vi "FGV Interference.vi"(0 "TestKonfig":T5={"CH4:"=0, "Ethane:"=0, "NMHC:"=0, "NMNEHC:"=0, "Komp 1 aktiv:"=FALSE, "Komp 2 aktiv:"=FALSE, "Komp 3 aktiv:"=FALSE, "Komp 4 aktiv:"=FALSE, "Modus"=0, "CG Aufschaltzeit:"=120.0, "Interferent 1: CO2"=0, "Interferent 2: H2O"=0, "Interferent 3: CH4"=0, "Interferent 4: C2H6 / C3H8"=0, "Gasflaschen Nr.:"="", "Gasflaschen Nr.: 3"="", "Gasflaschen Nr.: 4"="", "Inter 1 aktiv"=FALSE, "Inter 2 aktiv"=FALSE, "Inter 3 aktiv"=FALSE, "Inter 4 aktiv"=FALSE, "Accuracy"="", "Accuracy 3"="", "Accuracy 4"="", "Konzentration 1:"=120.0, "Konzentration 2:"=120.0, "Konzentration 3:"=120.0, "Konzentration 4:"=120.0, "Flow weighted mean 1:"=0.0, "Flow weighted mean 2:"=0.0, "Flow weighted mean 3:"=0.0, "Flow weighted mean 4:"=0.0} {"Flow weighted mean 4:" min=0.0; "Flow weighted mean 3:" min=0.0; "Flow weighted mean 2:" min=0.0; "Flow weighted mean 1:" min=0.0; "Konzentration 4:" min=0.0; "Konzentration 3:" min=0.0; "Konzentration 2:" min=0.0; "Konzentration 1:" min=0.0; "Modus" items=["Messen", "CG zu Entnahmestelle"]; "CG Aufschaltzeit:" min=60.0}, 1 "TestSetting":T1={"Bearbeiter:"="", "Pfad:"=path "D:/IAG_Data/Log", "Textname:"="", "Analysator"=""}, 5 "Ergebnis":sgl[](array[numeric]), 7 "Êinheiten":string[](array[string]), 9 "Tabelle":T3[][](array[typedef]), 11 "error in (no error)":errorcluster caption="Fehler (Eingang, kein Fehler)", 12 "Aktion FGV Interference":T7) -> (3 "TestSetting":T1={"Bearbeiter:"="", "Pfad:"=path "D:/IAG_Data/Log", "Textname:"="", "Analysator"=""}, 4 "TestKonfig":T5={"CH4:"=0, "Ethane:"=0, "NMHC:"=0, "NMNEHC:"=0, "Komp 1 aktiv:"=FALSE, "Komp 2 aktiv:"=FALSE, "Komp 3 aktiv:"=FALSE, "Komp 4 aktiv:"=FALSE, "Modus"=0, "CG Aufschaltzeit:"=120.0, "Interferent 1: CO2"=0, "Interferent 2: H2O"=0, "Interferent 3: CH4"=0, "Interferent 4: C2H6 / C3H8"=0, "Gasflaschen Nr.:"="", "Gasflaschen Nr.: 3"="", "Gasflaschen Nr.: 4"="", "Inter 1 aktiv"=FALSE, "Inter 2 aktiv"=FALSE, "Inter 3 aktiv"=FALSE, "Inter 4 aktiv"=FALSE, "Accuracy"="", "Accuracy 3"="", "Accuracy 4"="", "Konzentration 1:"=120.0, "Konzentration 2:"=120.0, "Konzentration 3:"=120.0, "Konzentration 4:"=120.0, "Flow weighted mean 1:"=0.0, "Flow weighted mean 2:"=0.0, "Flow weighted mean 3:"=0.0, "Flow weighted mean 4:"=0.0} {"Flow weighted mean 4:" min=0.0; "Flow weighted mean 3:" min=0.0; "Flow weighted mean 2:" min=0.0; "Flow weighted mean 1:" min=0.0; "Konzentration 4:" min=0.0; "Konzentration 3:" min=0.0; "Konzentration 2:" min=0.0; "Konzentration 1:" min=0.0; "Modus" items=["Messen", "CG zu Entnahmestelle"]; "CG Aufschaltzeit:" min=60.0}, 6 "Ergebnis":T4, 8 "Êinheiten":string[](array[string]), 10 "Tabelle":T3[][](array[typedef]), 15 "error out":errorcluster caption="Fehler (Ausgang)")   [LabVIEW 2020, in "EPA 1065.lvlib" / "Interference verificaton 1065-366.lvlib"]
uses:
  Interference verificaton 1065-366.lvlib
  Aktion FGV Interference.ctl
  TestKonfig.ctl
  Modus.ctl
  Ergebnis.ctl
  Visualisierungs Elemente/String - Ausgabefeld.ctl
  TestSetting.ctl
  Seiten/System Einstellungen V2/Analysatoren.ctl
  Linearisierung V2/AktivButton.ctl
  Allgemein/allgemeine Sub-VIs.lvlib
  Linearisierung V2/Linearisierung v2.lvlib
  Seiten/System Einstellungen V2/System Einstellungen V2.lvlib
panel:
  in  "Ergebnis":T4 caption="Cluster"
  # "sec."
  # "sec."
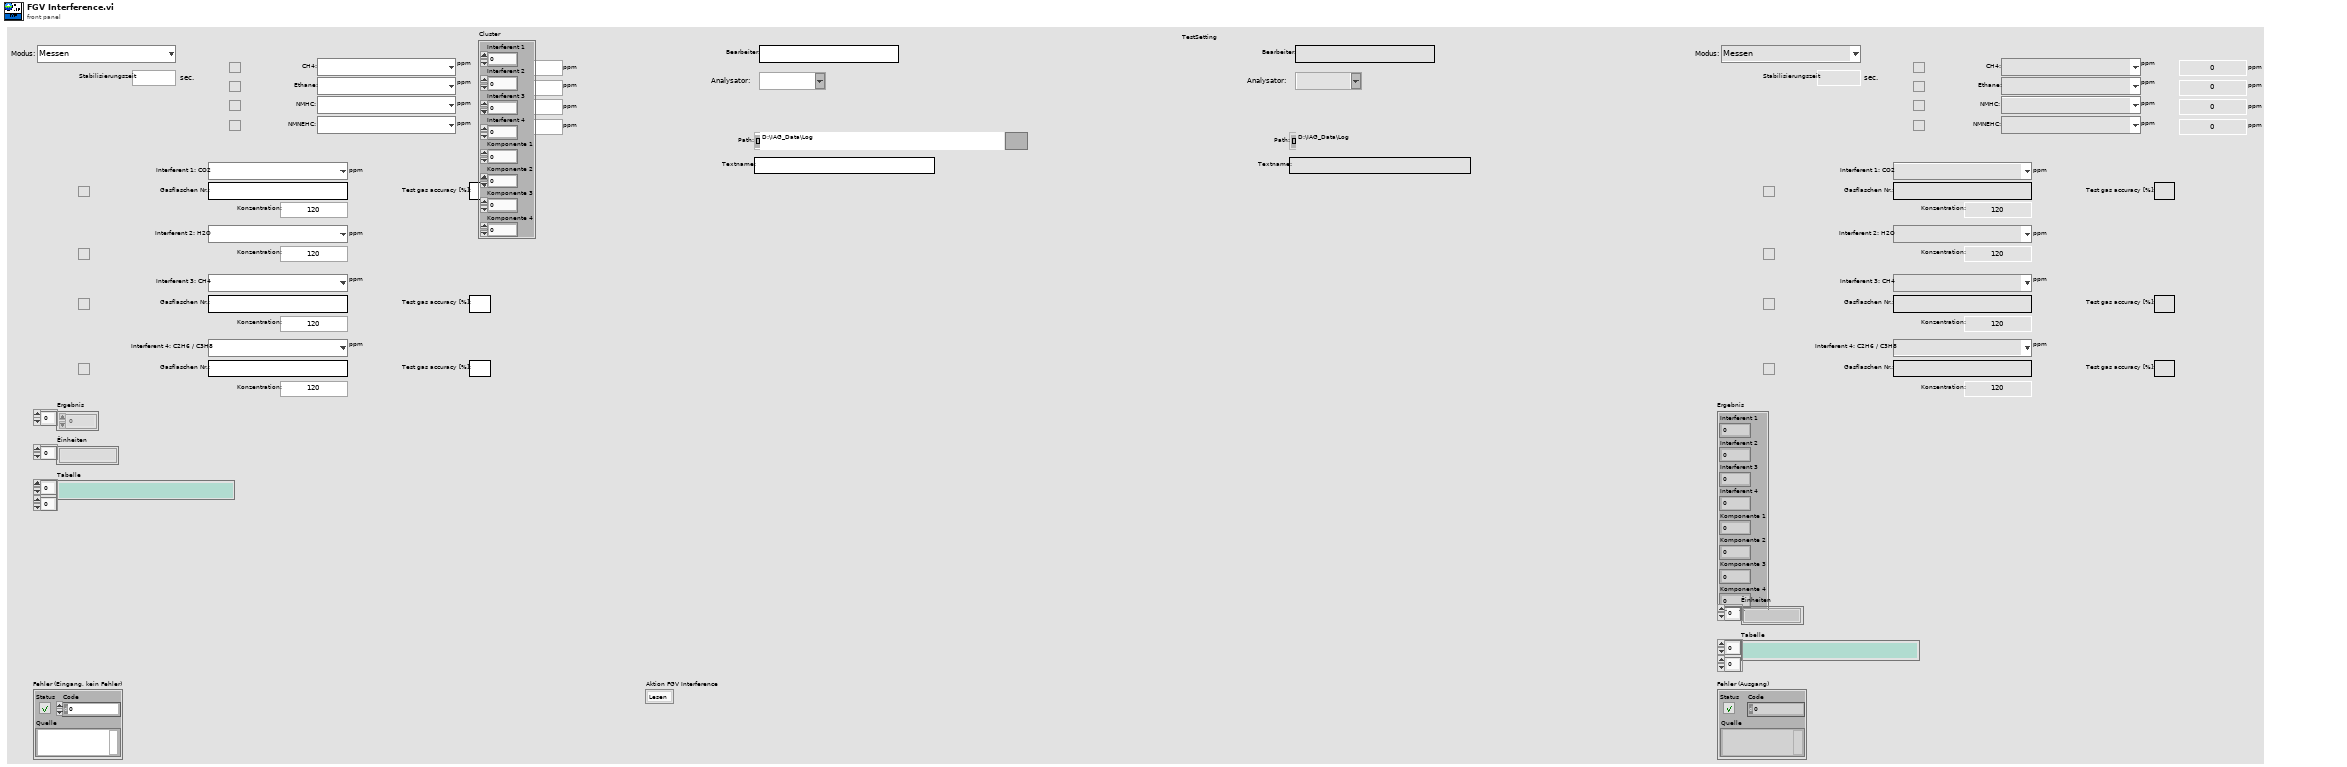
[diagram p1: front panel]
types:
  T1 = typedef "EPA 1065.lvlib/Interference verificaton 1065-366.lvlib/TestSetting.ctl" = cluster{"Bearbeiter:":string, "Pfad:":path, "Textname:":string, "Analysator":T2}
  T2 = typedef "System Einstellungen V2.lvlib/Analysatoren.ctl" = string
  T3 = typedef "String - Ausgabefeld.ctl" = string
  T4 = typedef "EPA 1065.lvlib/Interference verificaton 1065-366.lvlib/Ergebnis.ctl" = cluster{"Interferent 1":sgl, "Interferent 2":sgl, "Interferent 3":sgl, "Interferent 4":sgl, "Komponente 1":sgl, "Komponente 2":sgl, "Komponente 3":sgl, "Komponente 4":sgl}
  T5 = typedef "EPA 1065.lvlib/Interference verificaton 1065-366.lvlib/TestKonfig.ctl" = cluster{"CH4:":u16, "Ethane:":u16, "NMHC:":u16, "NMNEHC:":u16, "Komp 1 aktiv:":bool, "Komp 2 aktiv:":bool, "Komp 3 aktiv:":bool, "Komp 4 aktiv:":bool, "Modus":T6, "CG Aufschaltzeit:":dbl, "Interferent 1: CO2":u16, "Interferent 2: H2O":u16, "Interferent 3: CH4":u16, "Interferent 4: C2H6 / C3H8":u16, "Gasflaschen Nr.:":string, "Gasflaschen Nr.: 3":string, "Gasflaschen Nr.: 4":string, "Inter 1 aktiv":bool, "Inter 2 aktiv":bool, "Inter 3 aktiv":bool, "Inter 4 aktiv":bool, "Accuracy":string, "Accuracy 3":string, "Accuracy 4":string, "Konzentration 1:":dbl, "Konzentration 2:":dbl, "Konzentration 3:":dbl, "Konzentration 4:":dbl, "Flow weighted mean 1:":dbl, "Flow weighted mean 2:":dbl, "Flow weighted mean 3:":dbl, "Flow weighted mean 4:":dbl}
  T6 = typedef "EPA 1065.lvlib/Interference verificaton 1065-366.lvlib/Modus.ctl" = u16
  T7 = typedef "EPA 1065.lvlib/Interference verificaton 1065-366.lvlib/Aktion FGV Interference.ctl" = enum16{"Lesen", "TestKonfig", "TestSetting", "Einheiten", "Ergebnis", "Laden", "Tabelle", "Speichern", "löschen"}
  T8 = enum16{"open", "replace", "create", "open or create", "replace or create", "replace or create with confirmation"}
  T9 = typedef "Linearisierung v2.lvlib/AktivButton.ctl" = bool
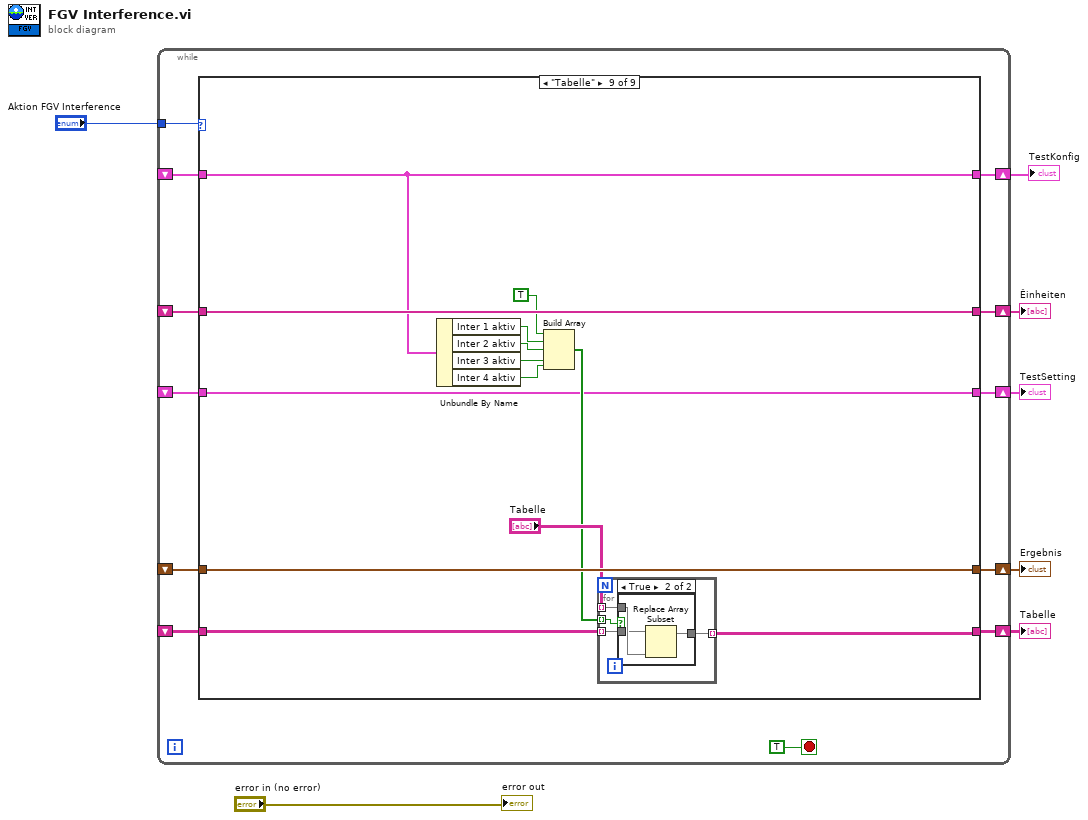
[diagram p0: block diagram]
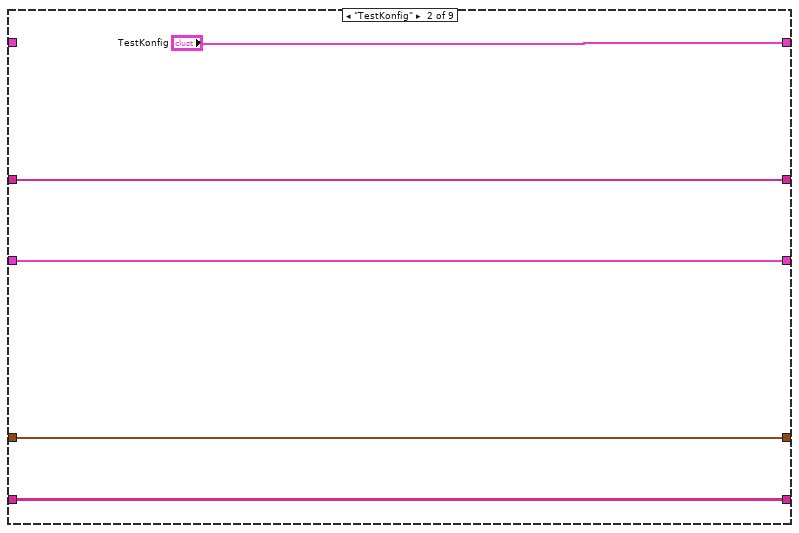
[diagram p3: hidden frame]
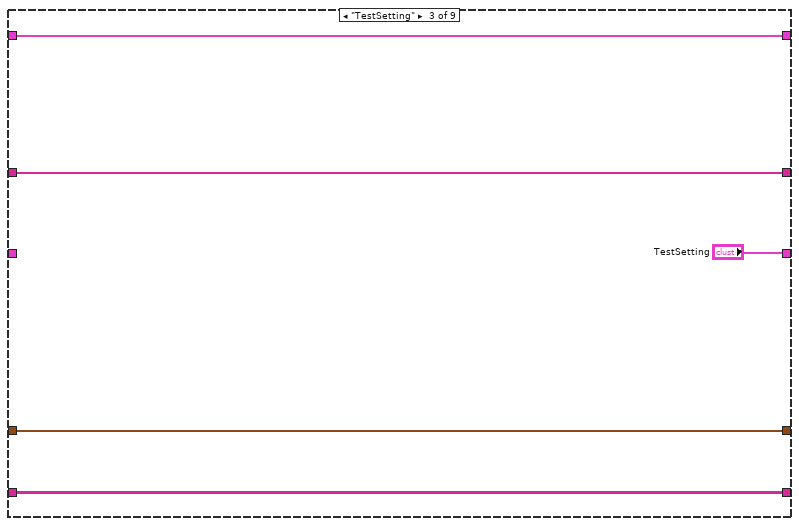
[diagram p4: hidden frame]
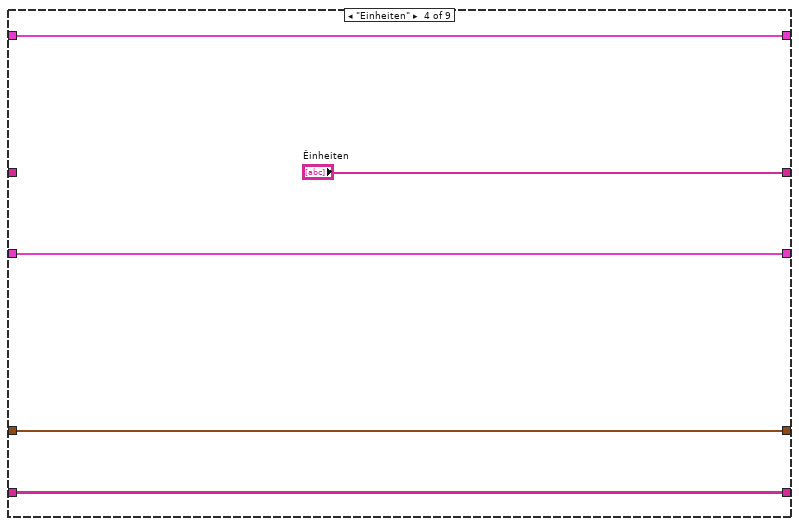
[diagram p5: hidden frame]
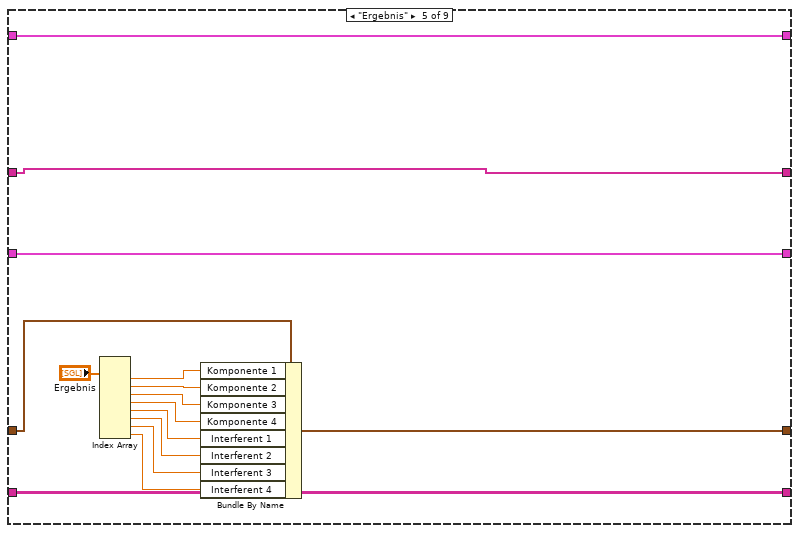
[diagram p6: hidden frame]
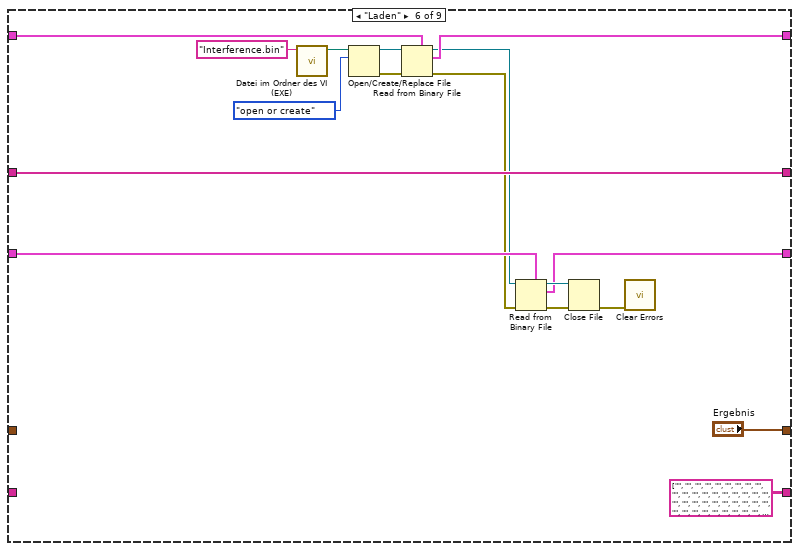
[diagram p7: hidden frame]
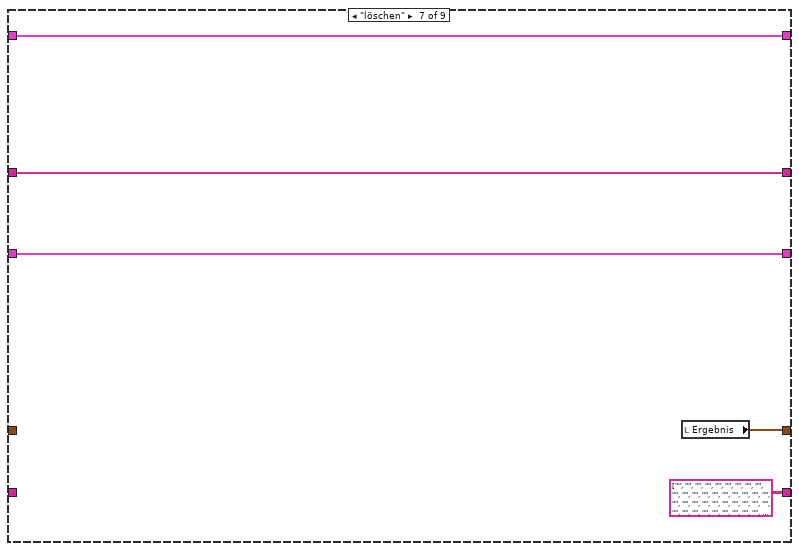
[diagram p8: hidden frame]
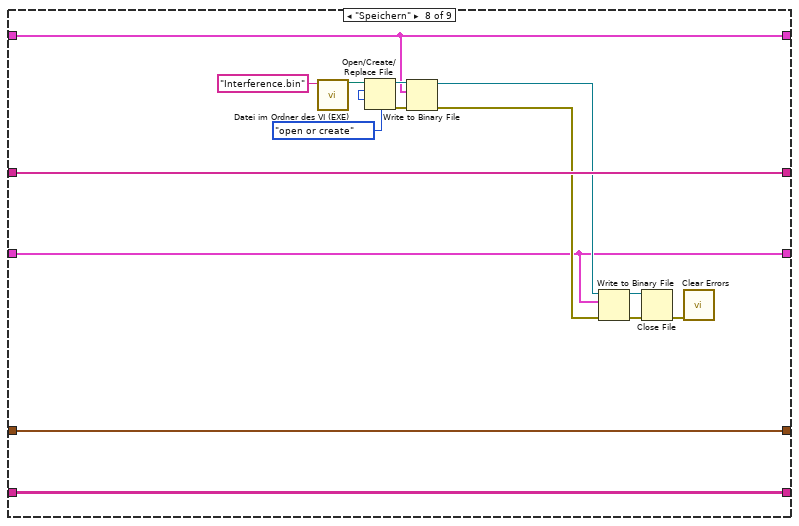
[diagram p9: hidden frame]
diagram:
  n1 = while {
    tunnel: "Aktion FGV Interference" -> [w18]
    shift-right: [w19] -> w5
    shift-left: _ -> [w17]
    shift-right: [w15] -> w4
    shift-left: _ -> [w14]
    shift-right: [w13] -> w3
    shift-left: _ -> [w12]
    shift-right: [w11] -> w2
    shift-left: _ -> [w10]
    shift-right: [w9] -> w1
    shift-left: _ -> [w8]
    stop <- TRUE stop-if-true
    n2 = case shown="\"Tabelle\"" w18 {
      tunnel: [w24 "TestKonfig" w31 w39 w54 w62 w74 w83 w102] -> w19
      tunnel: w17 -> [w24 _ w31 w39 w54 w63 w74 w83 w102]
      tunnel: [w23 w28 w34 w38 w46 "Ergebnis" w73 w91 w104] -> w15
      tunnel: w14 -> [w23 w28 w34 w38 w52 _ _ w91 w104]
      tunnel: [w22 w27 w33 "Êinheiten" w51 w70 w76 w90 w103] -> w13
      tunnel: w12 -> [w22 w27 w33 _ w51 w70 w76 w90 w103]
      tunnel: [w21 w26 w32 w36 w50 T3[][] [["", "", "", "", "", "", "", "", "", "", ""], ["", "", "", "", "", "", "", "", "", "", ""], ["", "", "", "", "", "", "", "", "", "", ""], ["", "", "", "", "", "", "", "", "", "", ""], ["", "", "", "", "", "", "", "", "", "", ""], ["", "", "", "", "", "", "", "", "", "", ""], ["", "", "", "", "", "", "", "", "", "", ""], ["", "", "", "", "", "", "", "", "", "", ""], ["", "", "", "", "", "", "", "", "", "", ""], ["", "", "", "", "", "", "", "", "", "", ""], ["", "", "", "", "", "", "", "", "", "", ""]] ("Tabelle") T3[][] [["", "", "", "", "", "", "", "", "", "", ""], ["", "", "", "", "", "", "", "", "", "", ""], ["", "", "", "", "", "", "", "", "", "", ""], ["", "", "", "", "", "", "", "", "", "", ""], ["", "", "", "", "", "", "", "", "", "", ""], ["", "", "", "", "", "", "", "", "", "", ""], ["", "", "", "", "", "", "", "", "", "", ""], ["", "", "", "", "", "", "", "", "", "", ""], ["", "", "", "", "", "", "", "", "", "", ""], ["", "", "", "", "", "", "", "", "", "", ""], ["", "", "", "", "", "", "", "", "", "", ""]] ("Tabelle") w89 w99] -> w11
      tunnel: w10 -> [w21 w26 w32 w36 w50 _ _ w89 w100]
      tunnel: [w20 w25 "TestSetting" w35 w45 w57 w72 w77 w92] -> w9
      tunnel: w8 -> [w20 w25 _ w35 w45 w58 w72 w77 w92]
      frame "Lesen", Default {
      }
      frame "TestKonfig" {
      }
      frame "TestSetting" {
      }
      frame "Einheiten" {
      }
      frame "Ergebnis" {
        n3 = Index Array(array="Ergebnis") -> (element #1=w49:sgl, element #2=w48:sgl, element #3=w47:sgl, element #4=w44:sgl, element #5=w43:sgl, element #6=w42:sgl, element #7=w41:sgl, element #8=w40:sgl)  [unwired: 8 in]
        n4 = Bundle By Name(cluster=w52, "Komponente 1"=w49, "Komponente 2"=w48, "Komponente 3"=w47, "Komponente 4"=w44, "Interferent 1"=w43, "Interferent 2"=w42, "Interferent 3"=w41, "Interferent 4"=w40) -> (w46:T4)
      }
      frame "Laden" {
        n5 = call "Datei im Ordner des VI (EXE).vi"("Dateiname"="Interference.bin") -> ("Dateipfad im Ordner des Haupt-VIs"=w67:path)  [unwired: 8 in, 2 out]
        n6 = Open/Create/Replace File(file path (use dialog)=w67, operation (0:open)=T8."open or create" ("Operation (0:open)")) -> (refnum out=w65:refnum<file>, error out=w66:errorcluster)  [unwired: 4 in, 1 out]
        n7 = Read from Binary File(5:w63, 8:w66, 11:w65) -> (0:w55:errorcluster, 2:w62:T5, 3:w56:refnum<file>)  [unwired: 3 in, 1 out]
        n8 = Read from Binary File(5:w58, 8:w55, 11:w56) -> (0:w59:errorcluster, 2:w57:T1, 3:w61:refnum<file>)  [unwired: 3 in, 1 out]
        n9 = Close File(refnum=w61, error in=w59) -> (error out=w60:errorcluster)  [unwired: 1 out]
        n10 = call <vilib>:"Clear Errors.vi"("error in (no error)"=w60) -> ()  [unwired: 5 in, 2 out]
      }
      frame "löschen" {
        n11 = local read "Ergebnis"() -> (w73:T4)
      }
      frame "Speichern" {
        n12 = call "Datei im Ordner des VI (EXE).vi"("Dateiname"="Interference.bin") -> ("Dateipfad im Ordner des Haupt-VIs"=w87:path)  [unwired: 8 in, 2 out]
        n13 = Open/Create/Replace File(file path (use dialog)=w87, operation (0:open)=T8."open or create" ("Operation (0:open)")) -> (refnum out=w88:refnum<file>, error out=w86:errorcluster)  [unwired: 4 in, 1 out]
        n14 = Write to Binary File(file (use dialog)=w88, data=w83, error in=w86) -> (refnum out=w79:refnum<file>, error out=w78:errorcluster)  [unwired: 3 in, 1 out]
        n15 = Write to Binary File(file (use dialog)=w79, data=w77, error in=w78) -> (refnum out=w81:refnum<file>, error out=w82:errorcluster)  [unwired: 3 in, 1 out]
        n16 = Close File(refnum=w81, error in=w82) -> (error out=w80:errorcluster)  [unwired: 1 out]
        n17 = call <vilib>:"Clear Errors.vi"("error in (no error)"=w80) -> ()  [unwired: 5 in, 2 out]
      }
      frame "Tabelle" {
        n18 = Unbundle By Name(w102) -> ("Inter 1 aktiv"=w98:bool, "Inter 2 aktiv"=w97:bool, "Inter 3 aktiv"=w96:bool, "Inter 4 aktiv"=w94:bool)
        n19 = Build Array(T9 TRUE ("Element"), w98, w97, w96, w94) -> (w95:T9[])
        n20 = for {
          tunnel: "Tabelle" -> [w108] mode=indexing
          tunnel: w100 -> [w107] mode=indexing
          tunnel: [w106] -> w99 mode=indexing
          tunnel: w95 -> [w105] mode=indexing
          n21 = case shown="True" w105 {
            tunnel: w108 -> [_ w112]
            tunnel: w107 -> [w109 w111]
            tunnel: [w109 w110] -> w106
            frame False {
            }
            frame True {
              n22 = Replace Array Subset(array=w111, new element=w112) -> (w110:T3[])  [unwired: 1 in]
            }
          }
        }
      }
    }
  }
  "TestKonfig" <- w5
  "Ergebnis" <- w4
  "Êinheiten" <- w3
  "Tabelle" <- w2
  "TestSetting" <- w1
  "error out" <- "error in (no error)"
